vi "MDOSave Data.vi"(7 "Data_save_directory":path, 8 "error in (no error)":errorcluster, 10 "Current Data":waveform(dbl)[](array[waveform]), 11 "Voltage Data":waveform(dbl)[](array[waveform])) -> (0 "error out":errorcluster)   [LabVIEW 2012]
doc: "Saves data to disk in the LVM file format."
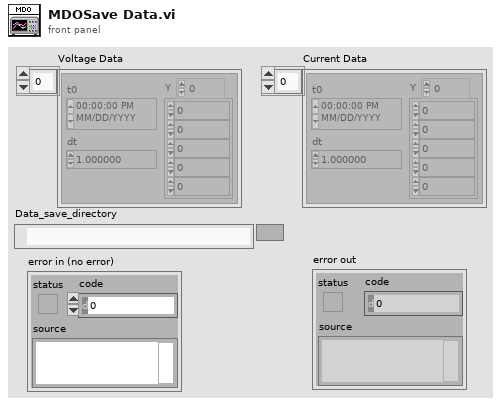
[diagram p1: front panel]
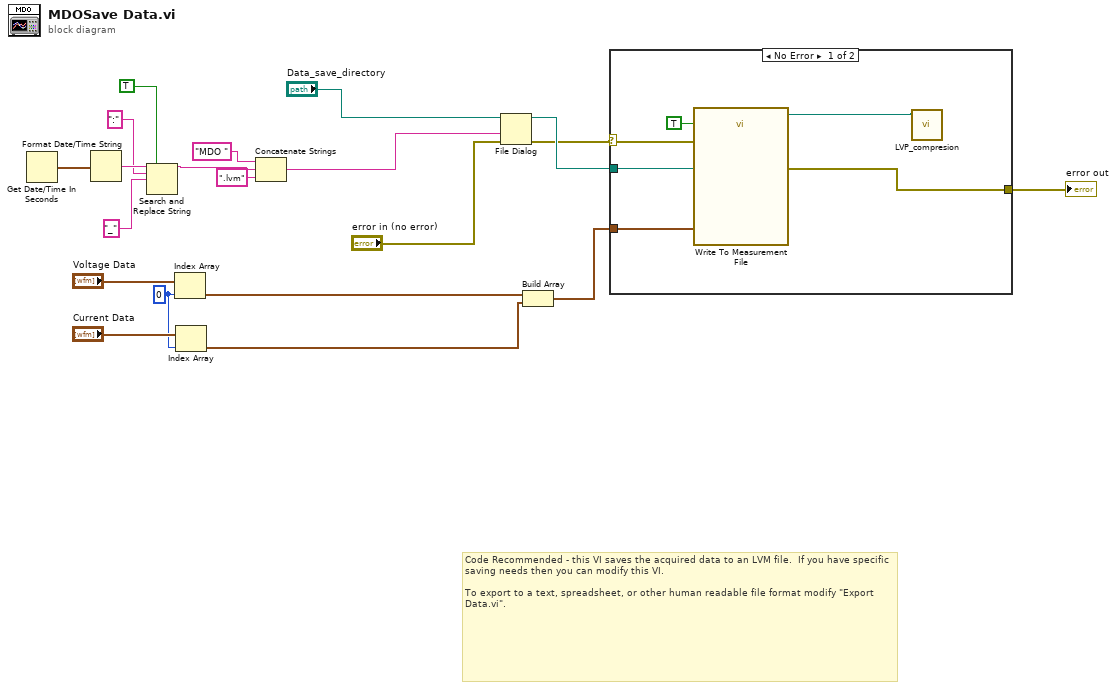
[diagram p0: block diagram]
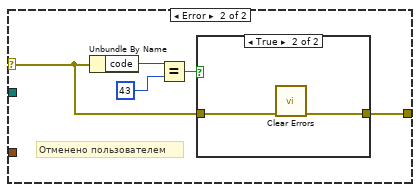
[diagram p2: hidden frame]
diagram:
  w18 = 0 ("index")
  # "Code Recommended - this VI saves the acquired data to an LVM file.  If you have specific saving needs then you can modify this VI.\n\nTo export to a text, spreadsheet, or other human readable file format modify \"Export Data.vi\"."
  n1 = Get Date/Time In Seconds() -> (seconds since 1Jan1904=w15:timestamp)
  n2 = Format Date/Time String(seconds (now)=w15) -> (date/time string=w13:string)  [unwired: 2 in]
  n3 = Search and Replace String(replace all?=TRUE ("replace all? (F)"), input string=w13, search string=":", replace string="_" ("replace string (\"\")")) -> (result string=w10:string)  [unwired: 4 in, 3 out]
  n4 = Index Array(array="Voltage Data", index=w18) -> (element=w5:waveform(dbl))
  n5 = Index Array(array="Current Data", index=w18) -> (element=w4:waveform(dbl))
  n6 = Concatenate Strings("MDO " ("string"), w10, ".lvm" ("string")) -> (w6:string)
  n7 = File Dialog(8:"error in (no error)", 9:w6, 11:"Data_save_directory") -> (0:w1:errorcluster, 3:w16:path)  [unwired: 4 in, 2 out]
  n8 = Build Array(w5, w4) -> (w3:waveform(dbl)[])
  n9 = case shown="No Error" w1 {
    selector: w1 -> [w21 w28]
    tunnel: w16 -> [w25 _]
    tunnel: w3 -> [w24 _]
    tunnel: [w23 w27] -> w2
    frame No Error {
      n10 = call "Write To Measurement File"("Signals"=w24, "Reset"=TRUE, "error in (no error)"=w21, "Filename"=w25) -> ("Filename Out"=w22:path, "error out"=w23:errorcluster)  [unwired: 13 in, 1 out]
      n11 = call "LVP_compresion.vi"("file path (dialog if empty)"=w22) -> ()  [unwired: 10 in, 1 out]
    }
    frame Error {
      # "Отменено пользователем"
      n12 = Unbundle By Name(w28) -> ("code"=w31:i32)
      n13 = Equal?(x=w31, y=43) -> (x = y?=w29:bool)
      n14 = case shown="True" w29 {
        tunnel: w28 -> [w32 w34]
        tunnel: [w32 w33] -> w27
        frame False {
        }
        frame True {
          n15 = call <vilib>:"Clear Errors.vi"("error in (no error)"=w34) -> ("error out"=w33:errorcluster)  [unwired: 6 in]
        }
      }
    }
  }
  "error out" <- w2
